vi "DC-Power Sequencer.vi"(0 "DCPower SSC in":T1[](array[typedef]), 1 "Voltage Level Range (V)":dbl format="%#_6p", 5 "Voltage Level Start":dbl, 7 "Voltage Stop":dbl, 9 "Voltage Step":dbl=1.0 min=1.0, 11 "error in":errorcluster, 12 "Source Delay (s)":dbl format="%#_6p") -> (4 "DCPower SSC out":T1[](array[typedef]), 15 "error out":errorcluster)   [LabVIEW 2019]
doc: "Sweep the voltage by using Sequence Source Mode. \nRemember to reset the Source Mode to Sequential after using this VI."
uses:
  Instrument Control/DCPower/SSC DCPower/SSC DCPower.ctl
  <instrlib>/niDCPower/nidcpower.llb/niDCPower Output Function.ctl
  <instrlib>/niDCPower/nidcpower.llb/niDCPower Source Mode.ctl
  <instrlib>/niDCPower/nidcpower.llb/niDCPower Wait For Event - Event.ctl
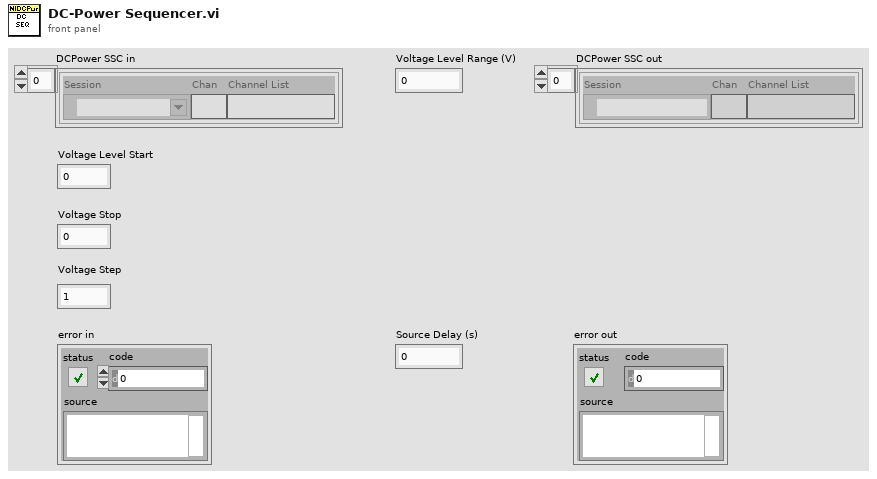
[diagram p1: front panel]
types:
  T1 = typedef "SSC DCPower.ctl" = cluster{"Session":refnum<k15>, "Chan":string, "Channel List":string}
  T2 = typedef "niDCPower Wait For Event - Event.ctl" = i32
  T3 = typedef "niDCPower Source Mode.ctl" = i32
  T4 = typedef "niDCPower Output Function.ctl" = i32
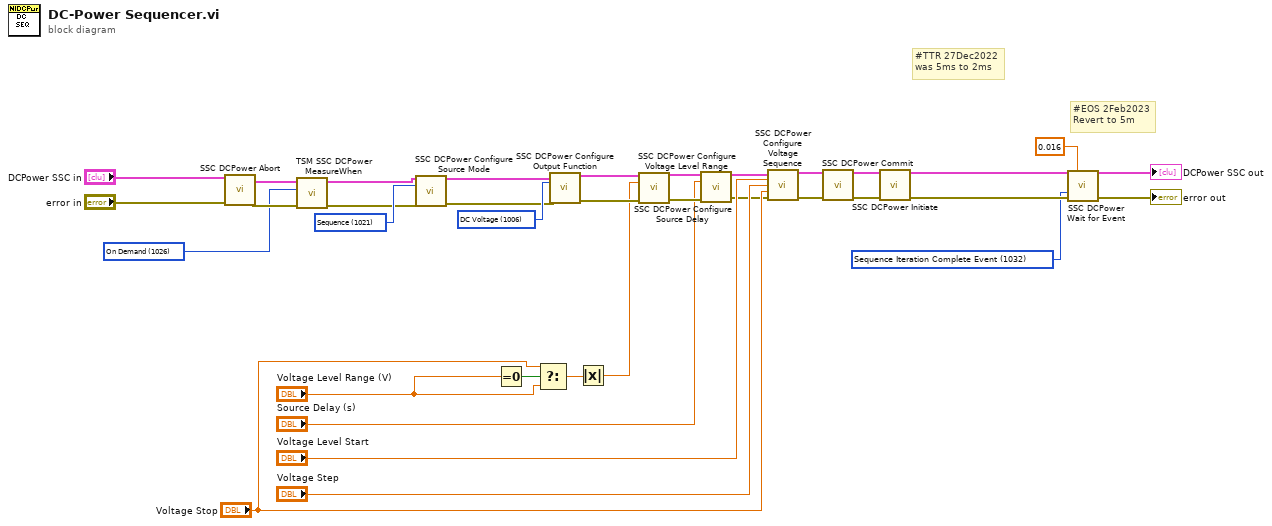
[diagram p0: block diagram]
diagram:
  w2 = 1026 items=["Automatically after Source Complete"=1025, "On Demand"=1026, "On Measure Trigger"=1027] ("Measurement:Advanced:Measure When")
  w8 = T2 1032 items=["Source Complete Event"=1030, "Measure Complete Event"=1031, "Sequence Iteration Complete Event"=1032, "Sequence Engine Done Event"=1033, "Pulse Complete Event"=1051, "Ready For Pulse Trigger Event"=1052] ("Event")
  w27 = T3 1021 items=["Single Point"=1020, "Sequence"=1021] ("Source Mode")
  w35 = T4 1006 items=["DC Voltage"=1006, "DC Current"=1007, "Pulse Voltage"=1049, "Pulse Current"=1050] ("Output Function")
  # "#EOS 2Feb2023\nRevert to 5m"
  # "#TTR 27Dec2022\nwas 5ms to 2ms"
  n1 = call "SSC DCPower Abort.vi"("DCPower SSC in"="DCPower SSC in", "error in"="error in") -> ("DCPower SSC out"=w6:T1[], "error out"=w5:errorcluster)  [unwired: 12 in]
  n2 = call "TSM SSC DCPower MeasureWhen.vi"("error in"=w5, "Measurement:Advanced:Measure When"=w2, "DCPower SSC in"=w6) -> ("error out"=w4:errorcluster, "DCPower SSC out"=w3:T1[])  [unwired: 7 in]
  n3 = call "SSC DCPower Configure Source Mode.vi"("DCPower SSC in"=w3, "Source Mode"=w27, "error in"=w4) -> ("DCPower SSC out"=w26:T1[], "error out"=w25:errorcluster)  [unwired: 11 in]
  n4 = Equal To 0?(x="Voltage Level Range (V)") -> (x = 0?=w30:bool)
  n5 = Select(t="Voltage Stop", s=w30, f="Voltage Level Range (V)") -> (s? t:f=w28:dbl)
  n6 = call "SSC DCPower Configure Output Function.vi"("DCPower SSC in"=w26, "Output Function"=w35, "error in"=w25) -> ("DCPower SSC out"=w11:T1[], "error out"=w12:errorcluster)  [unwired: 11 in]
  n7 = Absolute Value(x=w28) -> (abs(x)=w1:dbl)
  n8 = call "SSC DCPower Configure Voltage Level Range.vi"("DCPower SSC in"=w11, "Voltage Level Range (V)"=w1, "error in"=w12) -> ("DCPower SSC out"=w23:T1[], "error out"=w24:errorcluster)  [unwired: 11 in]
  n9 = call "SSC DCPower Configure Source Delay.vi"("DCPower SSC in"=w23, "Source Delay (s)"="Source Delay (s)", "error in"=w24) -> ("DCPower SSC out"=w21:T1[], "error out"=w10:errorcluster)  [unwired: 11 in]
  n10 = call "SSC DCPower Configure Voltage Sequence.vi"("DCPower SSC in"=w21, "Voltage Level Start"="Voltage Level Start", "Voltage Step"="Voltage Step", "Voltage Level Stop"="Voltage Stop", "error in"=w10) -> ("DCPower SSC out"=w20:T1[], "error out"=w19:errorcluster)  [unwired: 9 in]
  n11 = call "SSC DCPower Commit.vi"("DCPower SSC in"=w20, "error in"=w19) -> ("DCPower SSC out"=w31:T1[], "error out"=w32:errorcluster)  [unwired: 12 in]
  n12 = call "SSC DCPower Initiate.vi"("DCPower SSC in"=w31, "error in"=w32) -> ("DCPower SSC out"=w14:T1[], "error out"=w15:errorcluster)  [unwired: 12 in]
  n13 = call "SSC DCPower Wait for Event.vi"("DCPower SSC in"=w14, "Timeout (10s)"=0.016 ("Timeout"), "Event"=w8, "error in"=w15) -> ("DCPower SSC out"=→"DCPower SSC out":T1[], "error out"=→"error out":errorcluster)  [unwired: 10 in]
